vi "Express Vibration Lab.vi"() -> ()   [LabVIEW 2011, in "Sound and Vibration.lvclass"]
doc: "This application simulates a vibratory system of two masses and springs. You can control the system manually, automatically or by introducing generated signals. The parameters of the system, such as mass and rigidity of the springs can be changed. On the right side are graphs showing the values in the time and frequency domains.\n\nThis example uses the following Express VIs: Comparison, Formula, Repack Values, Spectral Measurements, Build XY Graph, and Simulate Signal."
uses:
  Sound and Vibration.lvclass
  Instance          11 29Saved   Express Vibration Lab .vi
  Instance           2 29Saved   Express Vibration Lab .vi
  Instance           1 29Saved   Express Vibration Lab .vi
  Instance           8 29Saved   Express Vibration Lab .vi
  Instance           3 29Saved   Express Vibration Lab .vi
  Instance          10 29Saved   Express Vibration Lab .vi
  <vilib>/express/express analysis/Spectral/Block/exnSpectralBlock spectral measurements peak poly.vi
  <vilib>/express/express analysis/Spectral/Block/exnSpectralBlock spectral measurements peak DDT.vi
  Instance           4 29Saved   Express Vibration Lab .vi
  Instance           5 29Saved   Express Vibration Lab .vi
  Instance           6 29Saved   Express Vibration Lab .vi
  Instance           7 29Saved   Express Vibration Lab .vi
  <vilib>/express/express arith-compare/Formula/XNode/ExpressFormulaBlockNode.xnode
  <vilib>/express/express analysis/Spectral/XNode/ExpressSpectralMeasurementsBlockNode.xnode
  Parent Plugin Definition/Plugin Template/Generic Plugin.lvclass
panel:
  in  "Rigidity 2":dbl=2.0 format="%0.2f"
  in  "Mass 2":dbl=1.0 format="%0.2f"
  in  "Mass 1":dbl=2.0 format="%0.2f"
  in  "Rigidity 1":dbl=8.0 format="%0.2f"
  in  "Generator Frequency":dbl(slide)=22.89156626506024 scale=0.0..100.0
  in  "Controller Type":i32(listbox)
  in  "Automatic P":dbl=6.0 format="%0.2f"
  in  "Automatic D":dbl=4.0 format="%0.2f"
  in  "Setpoint":dbl(slide) scale=-5.0..5.0
  in  "Manual":dbl(slide)=-2.822878228782288 scale=-5.0..5.0
  out "?":cluster{"Y":dbl[], "Y":dbl[]}[](graph)=[{"Y"=[0.0], "Y"=[0.0]}, {"Y"=[0.0], "Y"=[-5.0]}, {"Y"=[0.0], "Y"=[5.0]}, {"Y"=[0.5], "Y"=[0.0]}]
  out "Waveform Graph":dynamicdata(graph)=[{"t0"=timestamp(0 s since 1904-01-01), "dt"=inf, "Y"=[], "attributes"=variant("NI_ExpXDimension"=variant(string "f"))}, {"t0"=timestamp(0 s since 1904-01-01), "dt"=inf, "Y"=[], "attributes"=variant("NI_ExpXDimension"=variant(string "f"))}]
  out "Waveform Chart":dynamicdata(graph)=[{"t0"=timestamp(3096554047.203 s since 1904-01-01), "dt"=1.0, "Y"=[0.0]}, {"t0"=timestamp(3096554047.173 s since 1904-01-01), "dt"=1.0, "Y"=[0.0]}, {"t0"=timestamp(3096554047.243 s since 1904-01-01), "dt"=1.0, "Y"=[0.0]}, {"t0"=timestamp(3096554047.243 s since 1904-01-01), "dt"=1.0, "Y"=[0.0]}]
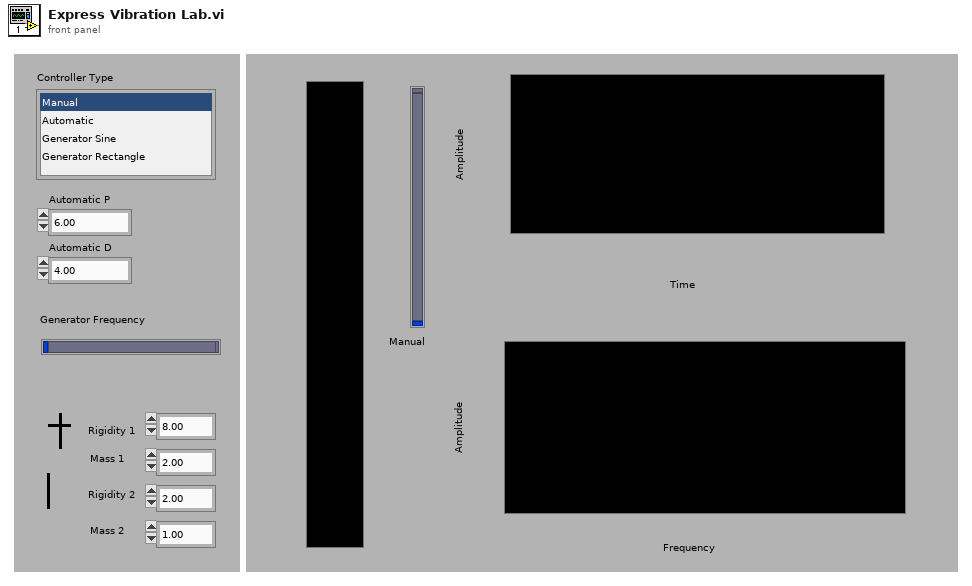
[diagram p1: front panel]
types:
  T1 = cluster{"averaging mode":u16, "weighting mode":u16, "number of averages":u32}
  T2 = cluster{"dB On (F)":bool, "unwrap phase (F)":bool, "convert to degree (F)":bool}
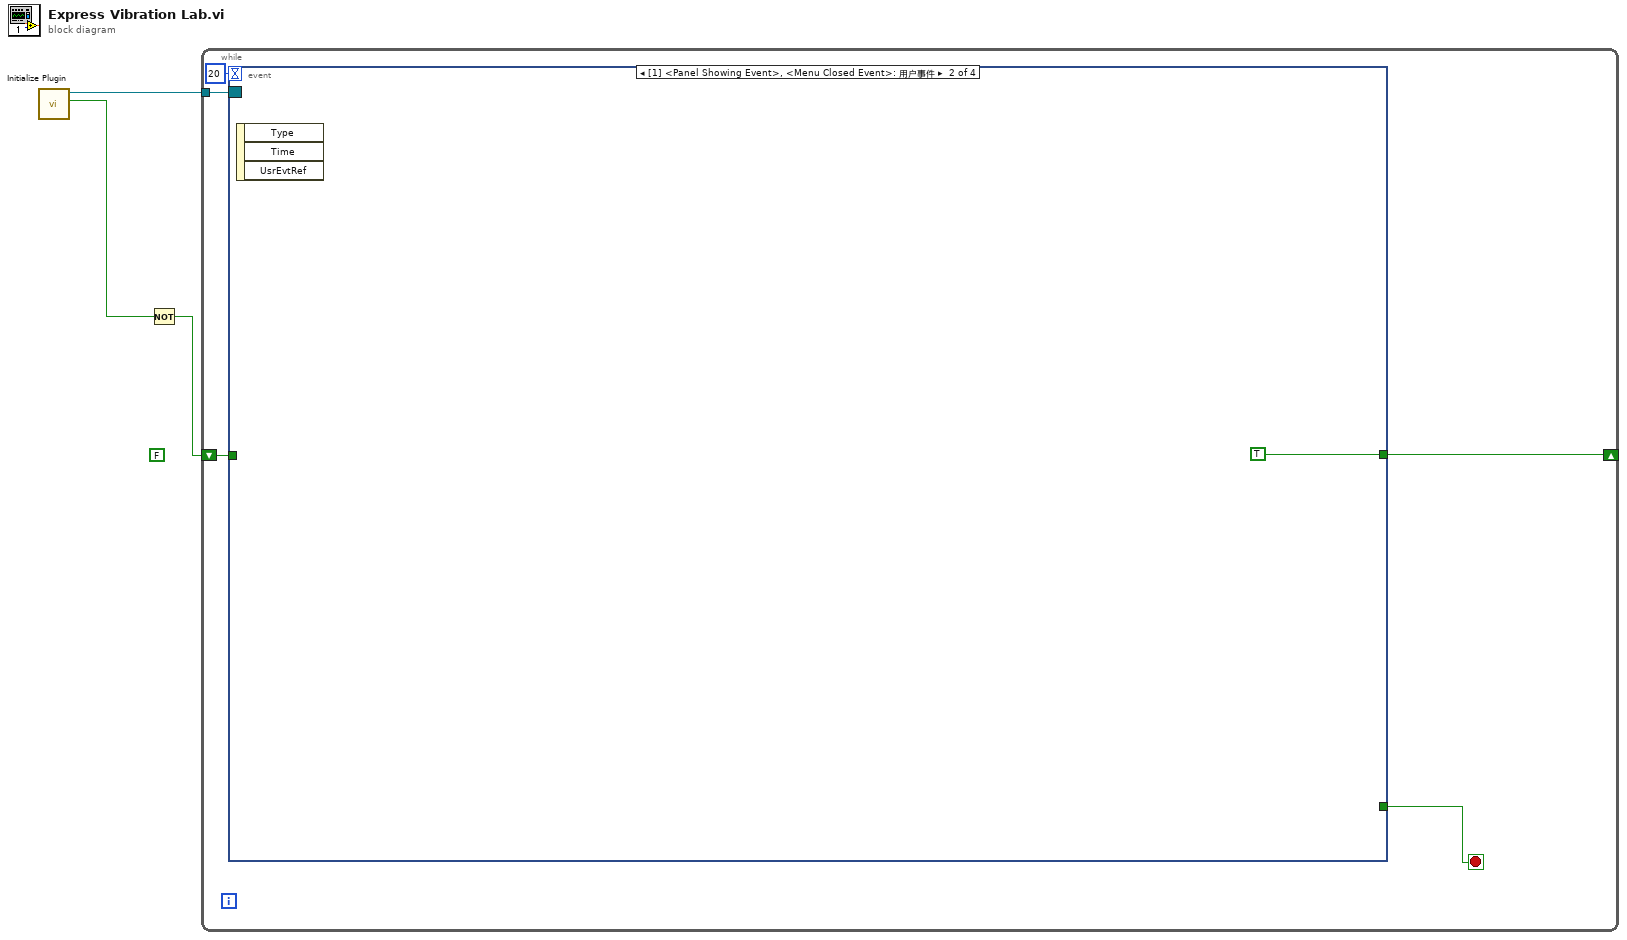
[diagram p0: block diagram]
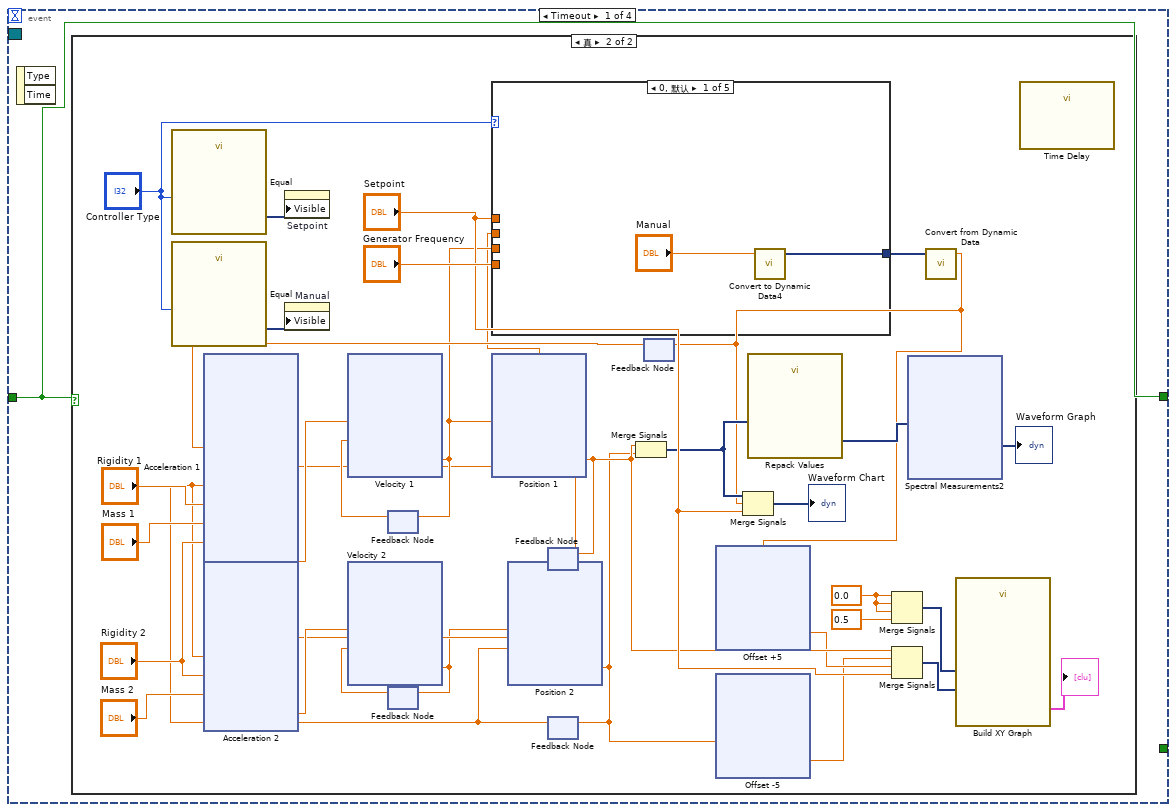
[diagram p2: hidden frame]
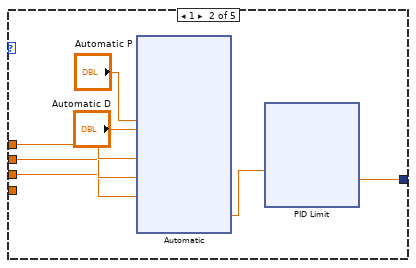
[diagram p4: hidden frame]
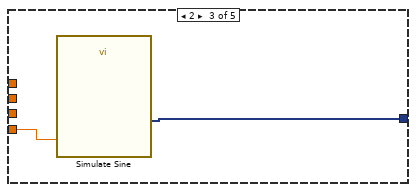
[diagram p5: hidden frame]
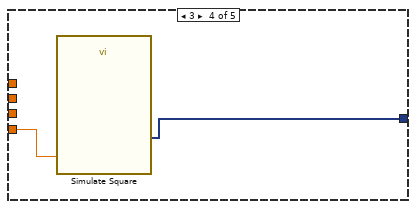
[diagram p6: hidden frame]
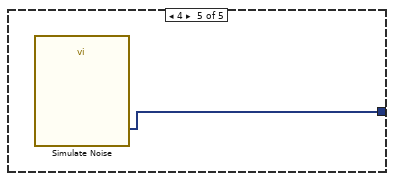
[diagram p7: hidden frame]
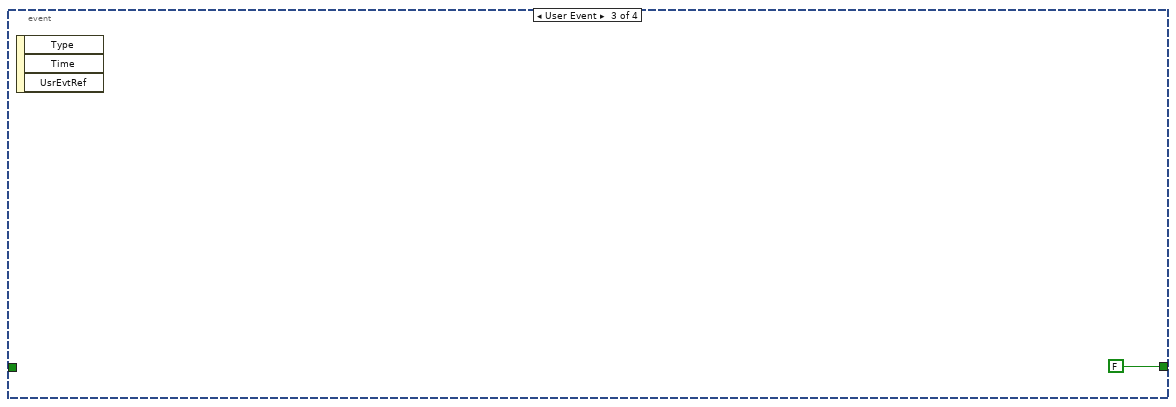
[diagram p8: hidden frame]
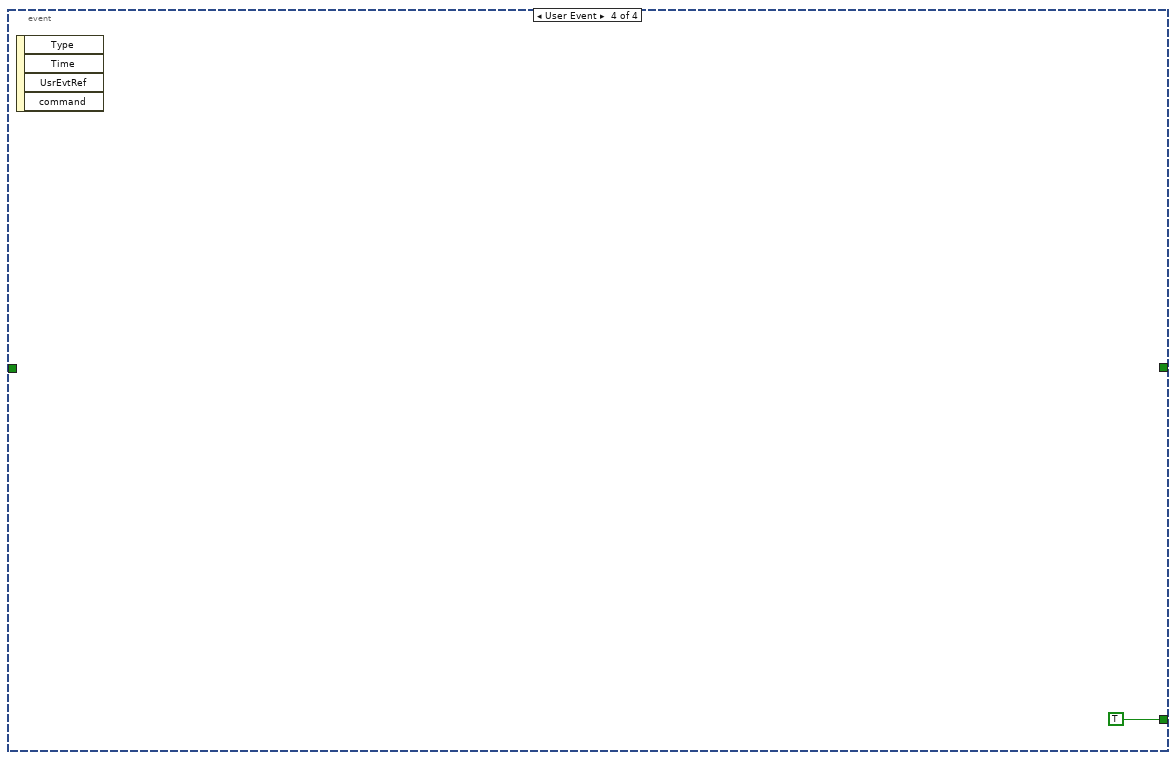
[diagram p9: hidden frame]
diagram:
  (unwired) FALSE
  n1 = call "Initialize Plugin.vi"() -> ("Called From Framework? Yes (T) No (F)"=w2:bool, "Event Registration Refnum"=w3:refnum<event-registration>)  [unwired: 9 in, 1 out]
  n2 = Not(x=w2) -> (.not. x?=w1:bool)
  n3 = while {
    tunnel: w3 -> [w7]
    shift-right: [w4] -> _
    shift-left: w1 -> [w5]
    stop <- w8 stop-if-true
    n4 = event shown="[1] <Panel Showing Event>, <Menu Closed Event>: 用户事件" {
      selector: w7 -> [_ _ _ _]
      dyn-events: _ -> [_ _ _ _]
      timeout: 20 -> [_ _ _ _]
      tunnel: [_ _ _ TRUE] -> w8
      tunnel: w5 -> [w9 _ _ _]
      tunnel: [w9 TRUE FALSE _] -> w4
      event Timeout {
        n5 = event-data() -> ()  [unwired: 1 in, 2 out]
        n6 = case shown="真" w9 {
          frame False {
          }
          frame True {
            w42 = 0.0
            n7 = call "Equal"("Operand 1"="Controller Type") -> ("Result"=w37:dynamicdata)  [unwired: 1 in, 9 out]
            n8 = call "Equal"("Operand 1"="Controller Type") -> ("Result"=w35:dynamicdata)  [unwired: 1 in, 9 out]
            n9 = property on="Setpoint" class="Slide (严格)"("Visible"=w37) -> ()  [unwired: 2 in, 2 out]
            n10 = property on="Manual" class="Slide (严格)"("Visible"=w35) -> ()  [unwired: 2 in, 2 out]
            n11 = feedback #1() -> (w21:dbl)  [unwired: 1 out]
            n12 = feedback #2() -> (w20:dbl)  [unwired: 1 out]
            n13 = feedback #3() -> (w17:dbl)  [unwired: 1 out]
            n14 = feedback #4() -> (w14:dbl)  [unwired: 1 out]
            n15 = xnode "Acceleration 2"("Position1"=w17, "Position2"=w14, "Rigidity2"="Rigidity 2", "Mass2"="Mass 2") -> ("结果"=w19:dbl)  [unwired: 1 in, 1 out]
            n16 = xnode "Velocity 2"("Accel"=w19, "Velocity"=w20) -> ("结果"=w15:dbl)  [unwired: 1 in, 1 out]
            n17 = feedback-in #2(w15) -> ()
            n18 = xnode "Position 2"("Velocity"=w15, "Position"=w14) -> ("结果"=w11:dbl)  [unwired: 1 in, 1 out]
            n19 = feedback-in #4(w11) -> ()
            n20 = feedback #5() -> (w27:dbl)  [unwired: 1 out]
            n21 = xnode "Acceleration 1"("Start"=w27, "Position1"=w17, "Position2"=w14, "Rigidity1"="Rigidity 1", "Mass1"="Mass 1", "Rigidity2"="Rigidity 2") -> ("结果"=w22:dbl)  [unwired: 1 in, 1 out]
            n22 = xnode "Velocity 1"("Accel"=w22, "Velocity"=w21) -> ("结果"=w18:dbl)  [unwired: 1 in, 1 out]
            n23 = feedback-in #1(w18) -> ()
            n24 = xnode "Position 1"("Velocity"=w18, "Position"=w17) -> ("结果"=w16:dbl)  [unwired: 1 in, 1 out]
            n25 = case shown="0, 默认" "Controller Type" {
              tunnel: w16 -> [_ w146 _ _ _]
              tunnel: w18 -> [_ w145 _ _ _]
              tunnel: "Setpoint" -> [_ w147 _ _ _]
              tunnel: [w141 w143 w174 w176 w178] -> w34
              tunnel: "Generator Frequency" -> [_ _ w175 w177 _]
              frame 0, Default {
                n26 = call "Convert to Dynamic Data4"("Double"="Manual") -> ("Dynamic Data Type"=w141:dynamicdata)  [unwired: 3 out]
              }
              frame 1 {
                n27 = xnode "Automatic"("P"="Automatic P", "D"="Automatic D", "setpoint"=w147, "position1"=w146, "velocity1"=w145) -> ("结果"=w144:dbl)  [unwired: 1 in, 1 out]
                n28 = xnode "PID Limit"("X1"=w144) -> ("结果"=w143:dbl)  [unwired: 1 in, 1 out]
              }
              frame 2 {
                n29 = call "Simulate Sine"("Frequency"=w175) -> ("Sine"=w174:dynamicdata)  [unwired: 5 in, 9 out]
              }
              frame 3 {
                n30 = call "Simulate Square"("Frequency"=w177) -> ("Square"=w176:dynamicdata)  [unwired: 5 in, 9 out]
              }
              frame 4 {
                n31 = call "Simulate Noise"() -> ("DC with Uniform Noise"=w178:dynamicdata)  [unwired: 5 in, 10 out]
              }
            }
            n32 = feedback-in #3(w16) -> ()
            n33 = Merge Signals(w16, w11) -> (w33:dynamicdata)
            n34 = xnode "Offset -5"("X1"=w11) -> ("结果"=w10:dbl)  [unwired: 1 in, 1 out]
            n35 = call "Repack Values"("Signals"=w33) -> ("Result"=w32:dynamicdata)  [unwired: 2 in, 8 out]
            n36 = Merge Signals(w42, w42, w42, 0.5) -> (w30:dynamicdata)
            n37 = xnode "Spectral Measurements2"("信号"=w32) -> ("FFT - (Peak)"=→"Waveform Graph":dynamicdata)  [unwired: 1 in, 2 out]
            n38 = call "Convert from Dynamic Data"("Dynamic Data Type"=w34) -> ("Scalar"=w13:dbl)  [unwired: 3 out]
            n39 = feedback-in #5(w13) -> ()
            n40 = xnode "Offset +5"("X1"=w13) -> ("结果"=w12:dbl)  [unwired: 1 in, 1 out]
            n41 = Merge Signals(w33, w13, "Setpoint") -> (→"Waveform Chart":dynamicdata)
            n42 = Merge Signals(w16, w10, w12, "Setpoint") -> (w29:dynamicdata)
            n43 = call "Build XY Graph"("Y Input"=w29, "X Input"=w30) -> ("XY Graph"=→"?":cluster{"Y":dbl[], "Y":dbl[]}[])  [unwired: 3 in, 6 out]
            n44 = call "Time Delay"() -> ()  [unwired: 2 in, 10 out]
          }
        }
      }
      event User Event {
        n45 = event-data() -> ()  [unwired: 1 in, 3 out]
      }
      event User Event {
        n46 = event-data() -> ()  [unwired: 1 in, 3 out]
      }
      event User Event {
        n47 = event-data() -> ()  [unwired: 1 in, 4 out]
      }
    }
  }
